vi "Write Name Library File Path.vi"(10 "Name Library File Path":path, 11 "_Rename in":refnum<class "_Rename.lvclass">) -> (3 "_Rename out":refnum<class "_Rename.lvclass">)   [LabVIEW 2025, in "_Rename.lvlib" / "_Rename.lvclass"]
uses:
  _Rename.lvclass
  _Rename.lvclass/_Rename.ctl
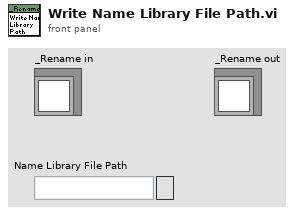
[diagram p1: front panel]
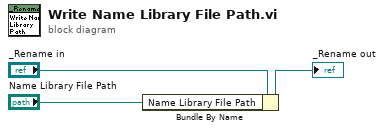
[diagram p0: block diagram]
diagram:
  n1 = Bundle By Name(cluster="_Rename in", "Name Library File Path"="Name Library File Path") -> (→"_Rename out":refnum<class "_Rename.lvclass">)
